vi "Test Find Two Separate Common Chars in Target.vi"(11 "Test Case In":refnum<class "Common Section Finder Test.lvclass">) -> (0 "error out":errorcluster, 3 "Test Case Out":refnum<class "Common Section Finder Test.lvclass">)   [LabVIEW 2020, in "Common Section Finder Test.lvclass"]
uses:
  Common Section Finder Test.lvclass
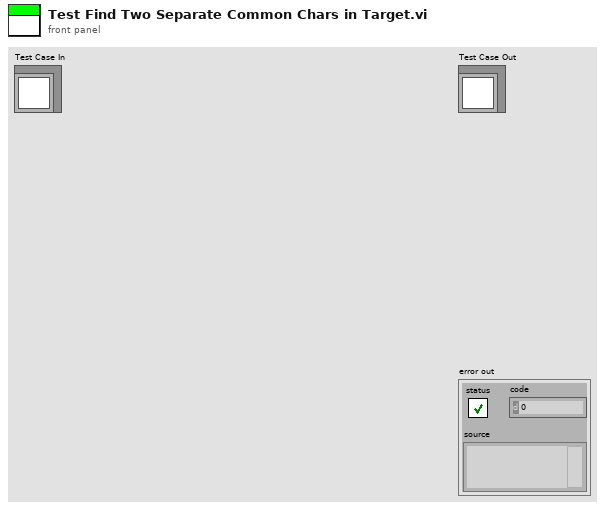
[diagram p1: front panel]
types:
  T1 = cluster{"Selection Start":i32, "Selection End":i32}
  T2 = cluster{"Selection Start":u32, "Selection End":u32}
  T3 = cluster{"Selection Start":u32, "Selection End":u32}[]
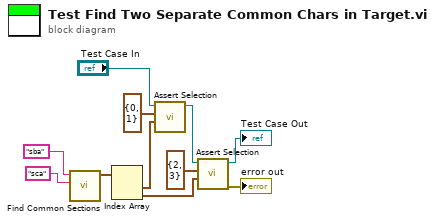
[diagram p0: block diagram]
diagram:
  n1 = call "Find Common Sections.vi"("Reference"="sca", "Target"="sba") -> ("Sections in Reference"=w8:T3)  [unwired: 9 in]
  n2 = Index Array(array=w8) -> (element #1=w6:T2, element #2=w1:T2)  [unwired: 2 in]
  n3 = call "Assert Selection.vi"("Actual"=w6, "Expected"=T2 {"Selection Start"=0, "Selection End"=1}, "Added Section Finder Test In"="Test Case In") -> ("Added Section Finder Test Out"=w5:refnum<class "Common Section Finder Test.lvclass">)  [unwired: 7 in, 1 out]
  n4 = call "Assert Selection.vi"("Actual"=w1, "Expected"=T1 {"Selection Start"=2, "Selection End"=3}, "Added Section Finder Test In"=w5) -> ("error out"=→"error out":errorcluster, "Added Section Finder Test Out"=→"Test Case Out":refnum<class "Common Section Finder Test.lvclass">)  [unwired: 7 in]
